vi "AddTerminal Char.vi"(4 "Cmd string":string) -> (1 "Concatenated String":string)   [LabVIEW 2025]
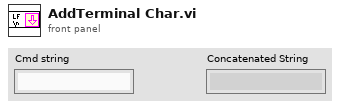
[diagram p1: front panel]
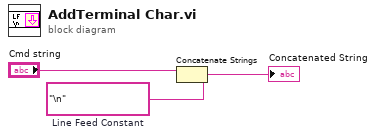
[diagram p0: block diagram]
diagram:
  w3 = "\n"  # Line Feed Constant
  n1 = Concatenate Strings("Cmd string", w3) -> (→"Concatenated String":string)
